vi "Drive Mode Cleaned.vi"   [LabVIEW 2017]
types:
  T1 = enum16{"Name Contains", "Name Equals", "HID Type", "XBox Type", "Axis Count", "Axis Type", "Button Count", "POV Count"}[]
  T2 = typedef "WPI_JoystickDeviceEnum.ctl" = enum16{"USB 0", "USB 1", "USB 2", "USB 3", "USB 4", "USB 5"}
  T3 = cluster{"[0]":bool, "[1]":bool, "[2]":bool, "[3]":bool, "[4]":bool, "[5]":bool, "[6]":bool, "[7]":bool, "[8]":bool}
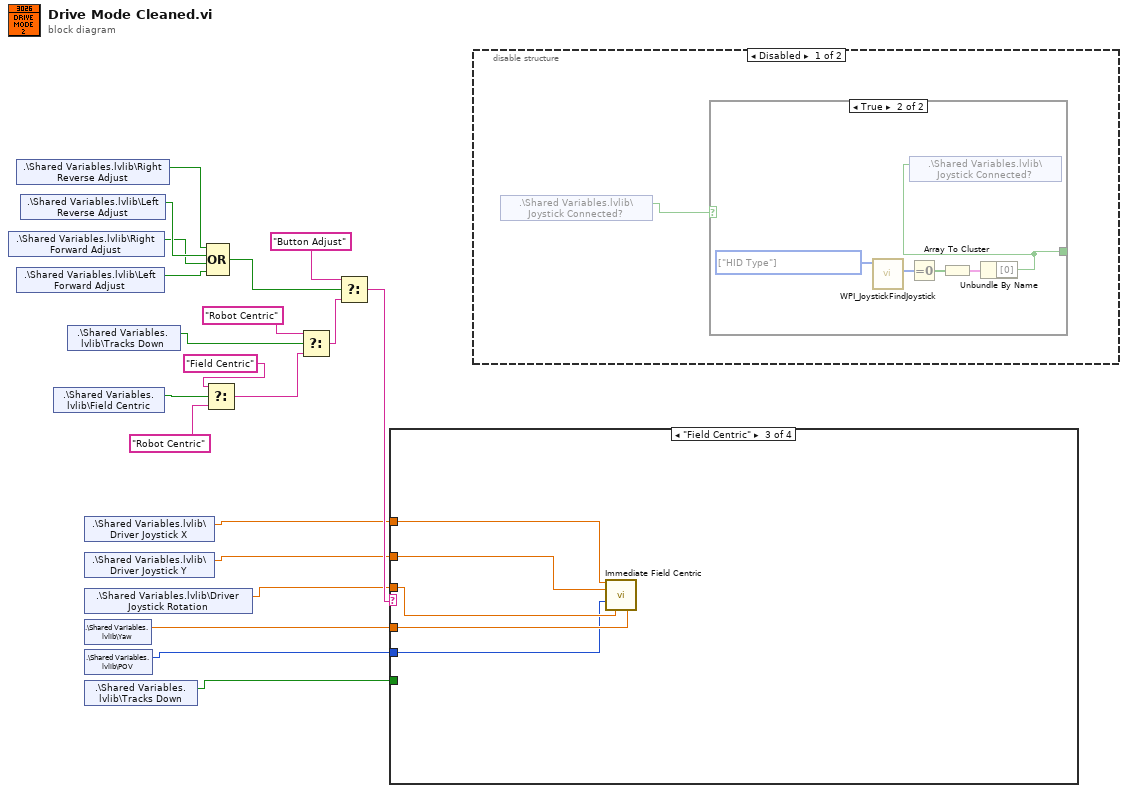
[diagram p0: block diagram]
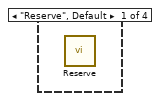
[diagram p4: hidden frame]
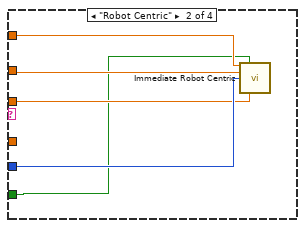
[diagram p5: hidden frame]
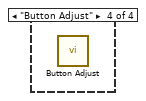
[diagram p6: hidden frame]
diagram:
  n1 = shared-variable ".\\Shared Variables.lvlib\\Right Forward Adjust"() -> (w3:bool)  [unwired: 1 in, 1 out]
  n2 = shared-variable ".\\Shared Variables.lvlib\\Right Reverse Adjust"() -> (w5:bool)  [unwired: 1 in, 1 out]
  n3 = shared-variable ".\\Shared Variables.lvlib\\Left Forward Adjust"() -> (w2:bool)  [unwired: 1 in, 1 out]
  n4 = shared-variable ".\\Shared Variables.lvlib\\Left Reverse Adjust"() -> (w4:bool)  [unwired: 1 in, 1 out]
  n5 = shared-variable ".\\Shared Variables.lvlib\\Field Centric"() -> (w19:bool)  [unwired: 1 in, 1 out]
  n6 = shared-variable ".\\Shared Variables.lvlib\\Tracks Down"() -> (w6:bool)  [unwired: 1 in, 1 out]
  n7 = shared-variable ".\\Shared Variables.lvlib\\Driver Joystick X"() -> (w15:dbl)  [unwired: 1 in, 1 out]
  n8 = shared-variable ".\\Shared Variables.lvlib\\Driver Joystick Y"() -> (w14:dbl)  [unwired: 1 in, 1 out]
  n9 = shared-variable ".\\Shared Variables.lvlib\\Driver Joystick Rotation"() -> (w13:dbl)  [unwired: 1 in, 1 out]
  n10 = shared-variable ".\\Shared Variables.lvlib\\Yaw"() -> (w12:dbl)  [unwired: 1 in, 1 out]
  n11 = shared-variable ".\\Shared Variables.lvlib\\POV"() -> (w11:i16)  [unwired: 1 in, 1 out]
  n12 = shared-variable ".\\Shared Variables.lvlib\\Tracks Down"() -> (w10:bool)  [unwired: 1 in, 1 out]
  n13 = Select(t="Field Centric", s=w19, f="Robot Centric") -> (s? t:f=w8:string)
  n14 = Compound Arithmetic op=OR(w5, w4, w3, w2) -> (w1:bool)
  n15 = Select(t="Robot Centric", s=w6, f=w8) -> (s? t:f=w9:string)
  n16 = Select(t="Button Adjust", s=w1, f=w9) -> (s? t:f=w16:string)
  n17 = case shown="\"Field Centric\"" w16 {
    tunnel: w15 -> [_ w25 w30 _]
    tunnel: w14 -> [_ w24 w29 _]
    tunnel: w13 -> [_ w22 w27 _]
    tunnel: w12 -> [_ _ w28 _]
    tunnel: w11 -> [_ w23 w26 _]
    tunnel: w10 -> [_ w21 _ _]
    frame "Reserve", Default {
      n18 = call "Reserve.vi"() -> ()  [unwired: 11 in, 1 out]
    }
    frame "Robot Centric" {
      n19 = call "Immediate Robot Centric.vi"("X Setpoint"=w25, "Tracks"=w21, "Y Setpoint"=w24, "POV"=w23, "Z Setpoint"=w22) -> ()  [unwired: 10 in, 1 out]
    }
    frame "Field Centric" {
      n20 = call "Immediate Field Centric.vi"("X Setpoint"=w30, "Y Setpoint"=w29, "POV"=w26, "Z Setpoint"=w27, "Gyro"=w28) -> ()  [unwired: 10 in, 1 out]
    }
    frame "Button Adjust" {
      n21 = call "Button Adjust.vi"() -> ()  [unwired: 11 in, 1 out]
    }
  }
  n22 = disable-structure shown="Disabled" {
    frame Disabled {
      n23 = shared-variable ".\\Shared Variables.lvlib\\Joystick Connected?"() -> (w31:bool)  [unwired: 1 in, 1 out]
      n24 = case shown="True" w31 {
        selector: w31 -> [w32 _]
        tunnel: [w32 w33] -> _
        frame False {
        }
        frame True {
          w37 = T1 [enum."HID Type"] items=["Name Contains", "Name Equals", "HID Type", "XBox Type", "Axis Count", "Axis Type", "Button Count", "POV Count"] ("Match Criteria")
          n25 = call <vilib>:"WPI_JoystickFindJoystick.vi"("Match Criteria"=w37) -> ("Matching Joysticks"=w36:T2[])  [unwired: 9 in, 1 out]
          n26 = Equal To 0?(x=w36) -> (x = 0?=w35:bool[])
          n27 = Array To Cluster(array=w35) -> (cluster=w34:T3)
          n28 = Unbundle By Name(w34) -> ("[0]"=w33:bool)
          n29 = shared-variable ".\\Shared Variables.lvlib\\Joystick Connected?"(w33) -> ()  [unwired: 1 in, 1 out]
        }
      }
    }
    frame Enabled {
    }
  }
